vi "Read Channel Voltage.vi"(11 "E3631A in":refnum<class "E3631A.lvclass">) -> (2 "Channel Voltage":dbl[](array[numeric]), 3 "E3631A out":refnum<class "E3631A.lvclass">)   [LabVIEW 2020, in "E3631A.lvclass"]
uses:
  E3631A.lvclass
  E3631A.lvclass/E3631A.ctl
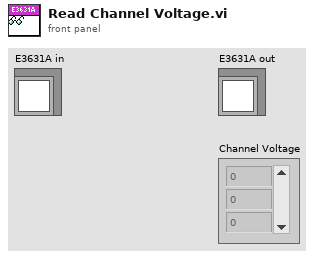
[diagram p1: front panel]
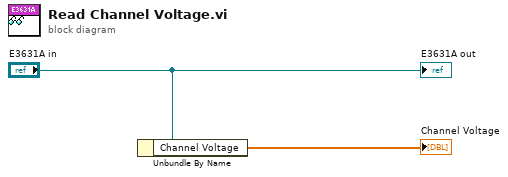
[diagram p0: block diagram]
diagram:
  n1 = Unbundle By Name("E3631A in") -> ("Channel Voltage"=→"Channel Voltage":dbl[])
  "E3631A out" <- "E3631A in"
